vi "Reduce Samples.vi"() -> ()   [LabVIEW 2015]
panel:
  out "Mean":dbl
  in  "Enable":bool=TRUE
  out "Sine":dynamicdata(graph)
  in  "stop":bool
  out "Table":string[][](table)
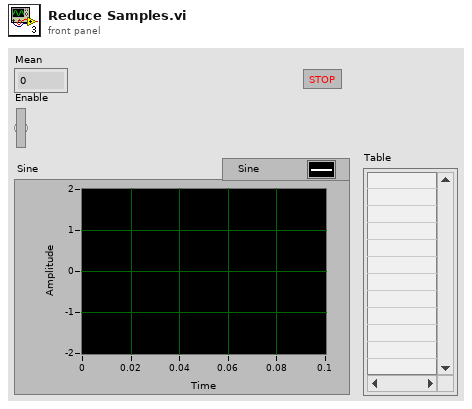
[diagram p1: front panel]
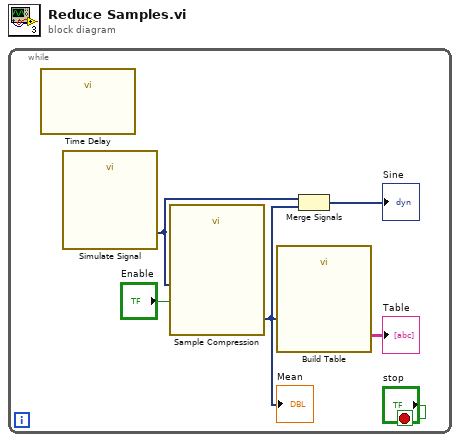
[diagram p0: block diagram]
diagram:
  n1 = while {
    stop <- "stop" stop-if-true
    n2 = call "Time Delay"() -> ()  [unwired: 11 in, 1 out]
    n3 = call "Simulate Signal"() -> ("Sine"=w6:dynamicdata)  [unwired: 14 in, 1 out]
    n4 = call "Sample Compression"("Enable"="Enable", "Signals"=w6) -> ("Mean"=w1:dynamicdata)  [unwired: 7 in, 2 out]
    "Mean" <- w1
    n5 = call "Build Table"("Signals"=w1) -> ("Table"=→"Table":string[][])  [unwired: 9 in, 1 out]
    n6 = Merge Signals(w6, w1) -> (→"Sine":dynamicdata)
  }
